vi "Freerun.vi"   [LabVIEW 2020, in "Aerotech VIs.lvlib"]
uses:
  Aerotech VIs.lvlib
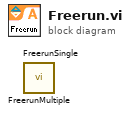
[diagram p0: block diagram]
diagram:
  n1 = call "FreerunMultiple.vi"() -> ()  [unwired: 10 in, 2 out]
  n2 = call "FreerunSingle.vi"() -> ()  [unwired: 10 in, 2 out]
